vi "SensorReadMove.vi"() -> ()   [LabVIEW 2016]
uses:
  Control/Control 1.ctl
  Other Models/2010/Status/AxisDiagPacket.ctl
  Other Models/2010/Status/ControllerDiagPacket.ctl
  <vilib>/Instr/_visa.llb/VISA Configure Serial Port (Instr).vi
panel:
  in  "Speed":dbl format="%#_13g"
  in  "baud rate":u32=115200
  in  "data bits":u16=8 min=5 max=8 step=1
  in  "parity":u16(ring)=2 items=["None", "Odd", "Even", "Mark", "Space"]
  in  "stop bits":u16(ring)=10 items=["1"=10, "1.5"=15, "2.0"=20]
  in  "flow control":u16(ring) items=["None"=0, "XON/XOFF"=1, "RTS/CTS"=2, "DTR/DSR"=4]
  in  "VISA resource name":refnum<visa-resource-name>="COM4"
  out "Boolean":bool=TRUE
  in  "Iterration":i32
  in  "Input2":cluster{"X":dbl, "Y":dbl}
  in  "Input1":cluster{"X":dbl, "Y":dbl}
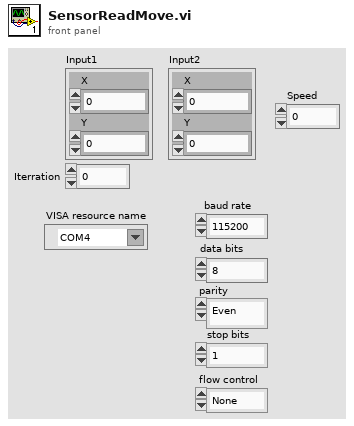
[diagram p1: front panel]
types:
  T1 = typedef "ControllerDiagPacket.ctl" = cluster{"Number of Diag Packets":i32, "Axes":T2[], "error":errorcluster}
  T2 = typedef "AxisDiagPacket.ctl" = cluster{"Axis Name":string, "Analog Input 0":dbl, "Analog Input 1":dbl, "Axis Fault (num)":i32, "Axis Fault (str)":string, "Axis Fault (bits)":cluster{"AmplifierFault":bool, "AmplifierTemperatureFault":bool, "CcwEndOfTravelLimitFault":bool, "CcwSoftwareLimitFault":bool, "CommunicationLostFault":bool, "CwEndOfTravelLimitFault":bool, "CwSoftwareLimitFault":bool, "EmergencyStopFault":bool, "EncoderFault":bool, "ExternalFault":bool, "FeedbackScalingFault":bool, "GantryMisalignFault ":bool, "HallSensorFault":bool, "InPositionTimeoutFault":bool, "InternalFault":bool, "MarkerSearchFault":bool, "MaxVelocityCommandFault":bool, "MissedInterruptFault":bool, "MotorTemperatureFault":bool, "None":bool, "OverCurrentFault":bool, "PositionErrorFault":bool, "PositionFeedbackFault":bool, "PowerSupplyFault":bool, "ProbeInputFault":bool, "SafeZoneFault":bool, "VelocityErrorFault":bool, "VelocityFeedbackFault":bool, "VoltageClampFault":bool}, "Axis Status (num)":i32, "Axis Status (str)":string, "Axis Status (bits)":cluster{"BacklashActive":bool, "CalibrationEnabled1D":bool, "CalibrationEnabled2D":bool, "CommandValid":bool, "DriveAbortPending":bool, "DrivePending":bool, "Enabling":bool, "GainMappingEnabled":bool, "GantryAligned":bool, "GantryRealigning":bool, "Homed":bool, "Homing":bool, "IFOVEnabled":bool, "JogGenerating":bool, "Jogging":bool, "JoystickControl":bool, "MasterSlaveControl":bool, "MotionBlocked":bool, "MotionClamped":bool, "MoveDone":bool, "None":bool, "NotVirtual":bool, "Profiling":bool, "Stability0":bool, "Stability1":bool, "TrajectoryFiltering":bool, "WaitDone":bool}, "Current Command":sgl, "Current Error":sgl, "Current Feedback":sgl, "Digital Inputs":i32, "Digital Outputs":i32, "Drive Status":i32, "Drive Status (str)":string, "Drive Status (bits)":cluster{"AccelerationPhase":bool, "AutofocusActive":bool, "BrakeOutput":bool, "CcwEndOfTravelLimitInput":bool, "CosineEncoderError":bool, "CurrentClamp":bool, "CwEndOfTravelLimitInput":bool, "DecelerationPhase":bool, "DualLoopActive":bool, "EmergencyStopInput":bool, "Enabled":bool, "EncoderClipping":bool, "GalvoCalibrationEnabled":bool, "GalvoPowerCorrection":bool, "HallAInput":bool, "HallBInput":bool, "HallCInput":bool, "HighResolutionMode":bool, "HomeLimitInput":bool, "InPosition":bool, "InPosition2":bool, "MarkerInput":bool, "MarkerLatch":bool, "MoveActive":bool, "NoMotorSupply":bool, "None":bool, "PowerLimiting":bool, "ProgrammingFlash":bool, "ProgrammingMXH":bool, "PSOHaltLatch":bool, "ServoControl":bool, "SineEncoderError":bool}, "Position Feedback Auxiliary":dbl, "Position Command":dbl, "Position Error":dbl, "Position Feedback":dbl, "Program Position Command":dbl, "Program Position Error":dbl, "Program Position Feedback":dbl, "Velocity Command":dbl, "Velocity Error":dbl, "Velocity Feedback":dbl}
  T3 = typedef "Control 1.ctl" = string[]
  T4 = cluster{"ControllerDiagPacket":T1, "read buffer":string}
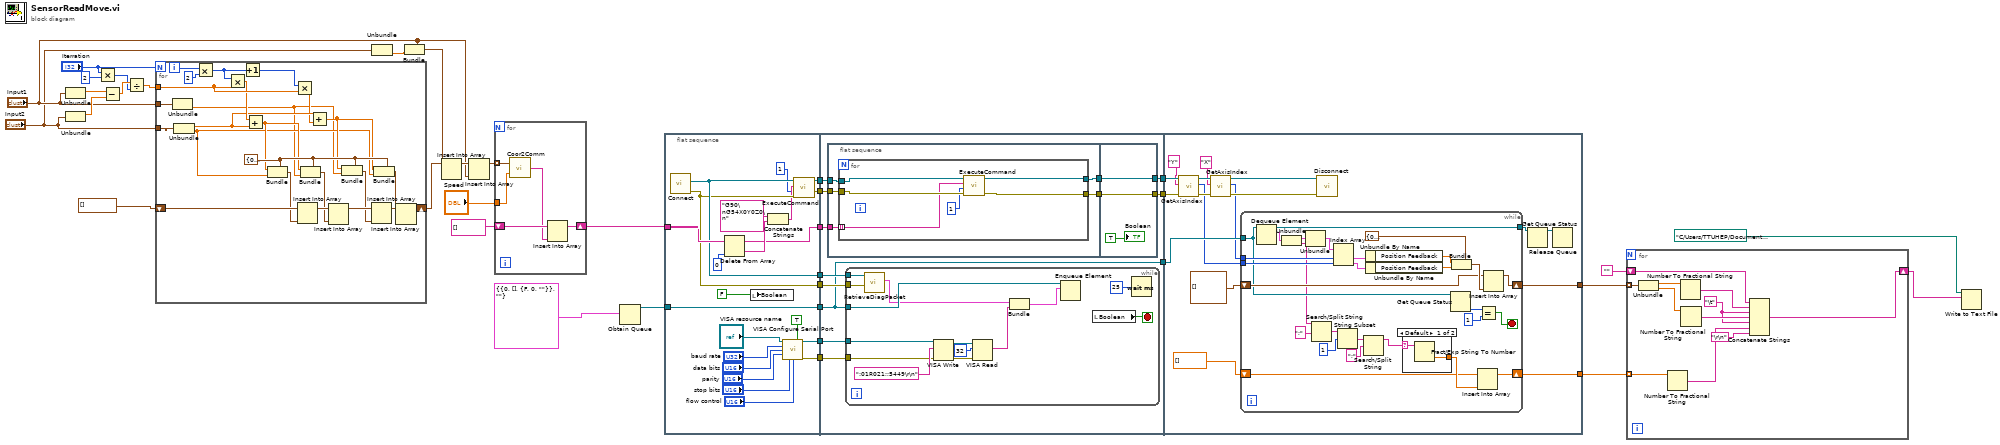
[diagram p0: block diagram]
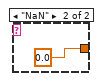
[diagram p2: hidden frame]
diagram:
  n1 = Unbundle("Input1") -> ("X"=w36:dbl)  [unwired: 1 out]
  n2 = Unbundle("Input2") -> ("X"=w35:dbl)  [unwired: 1 out]
  n3 = Multiply(x="Iterration", y=2) -> (x*y=w31:i32)
  n4 = Subtract(x=w36, y=w35) -> (x-y=w34:dbl)
  n5 = Divide(x=w34, y=w31) -> (x/y=w30:dbl)
  n6 = for {
    N: "Iterration" -> [_]
    tunnel: "Input1" -> [w49]
    tunnel: "Input2" -> [w50]
    tunnel: w30 -> [w46]
    shift-right: [w56] -> w26
    shift-left: cluster{"X":dbl, "Y":dbl}[] [] -> [w60]
    i -> [w39]
    w51 = cluster{"X":dbl, "Y":dbl} {"X"=0.0, "Y"=0.0}
    n7 = Unbundle(w49) -> ("Y"=w37:dbl)  [unwired: 1 out]
    n8 = Unbundle(w50) -> ("X"=w41:dbl, "Y"=w38:dbl)
    n9 = Multiply(x=w39, y=2) -> (x*y=w47:i32)
    n10 = Multiply(x=w47, y=w46) -> (x*y=w44:dbl)
    n11 = Increment(x=w47) -> (x+1=w45:i32)
    n12 = Add(x=w44, y=w41) -> (x+y=w43:dbl)
    n13 = Bundle(cluster=w51, "X"=w43, "Y"=w38) -> (w55:cluster{"X":dbl, "Y":dbl})
    n14 = Multiply(x=w45, y=w46) -> (x*y=w40:dbl)
    n15 = Insert Into Array(array=w60, new element=w55) -> (w59:cluster{"X":dbl, "Y":dbl}[])  [unwired: 1 in]
    n16 = Bundle(cluster=w51, "X"=w43, "Y"=w37) -> (w54:cluster{"X":dbl, "Y":dbl})
    n17 = Add(x=w41, y=w40) -> (x+y=w42:dbl)
    n18 = Insert Into Array(array=w59, new element=w54) -> (w58:cluster{"X":dbl, "Y":dbl}[])  [unwired: 1 in]
    n19 = Bundle(cluster=w51, "X"=w42, "Y"=w37) -> (w53:cluster{"X":dbl, "Y":dbl})
    n20 = Insert Into Array(array=w58, new element=w53) -> (w57:cluster{"X":dbl, "Y":dbl}[])  [unwired: 1 in]
    n21 = Bundle(cluster=w51, "X"=w42, "Y"=w38) -> (w52:cluster{"X":dbl, "Y":dbl})
    n22 = Insert Into Array(array=w57, new element=w52) -> (w56:cluster{"X":dbl, "Y":dbl}[])  [unwired: 1 in]
  }
  n23 = Unbundle("Input2") -> ("Y"=w20:dbl)  [unwired: 1 out]
  n24 = Bundle(cluster="Input1", "Y"=w20) -> (w23:cluster{"X":dbl, "Y":dbl})  [unwired: 1 in]
  n25 = Insert Into Array(array=w26, new element=w23) -> (w25:cluster{"X":dbl, "Y":dbl}[])  [unwired: 1 in]
  n26 = Insert Into Array(array=w25, new element="Input1") -> (w24:cluster{"X":dbl, "Y":dbl}[])  [unwired: 1 in]
  n27 = for {
    tunnel: w24 -> [w62] mode=indexing
    shift-right: [w64] -> w27
    shift-left: T3 [] -> [w65]
    tunnel: "Speed" -> [w61]
    n28 = call "Coor2Comm.vi"("Numeric"=w61, "Cluster"=w62) -> ("String"=w63:string)
    n29 = Insert Into Array(array=w65, new element=w63) -> (w64:T3)  [unwired: 1 in]
  }
  n30 = Obtain Queue(element data type=cluster{"ControllerDiagPacket":T1, string} {"ControllerDiagPacket"={"Number of Diag Packets"=0, "Axes"=[], "error"={"status"=FALSE, "code"=0, "source"=""}}, ""}) -> (queue out=w12:refnum<queue>)  [unwired: 4 in, 2 out]
  n31 = flat-sequence {
    tunnel: [w79] -> w17
    tunnel: [w83] -> w16
    tunnel: [w84] -> w15
    tunnel: w27 -> [w87]
    tunnel: [w86] -> w14
    tunnel: [w85] -> w13
    tunnel: w12 -> [w76]
    tunnel: [w76] -> w11
    tunnel: [w68] -> w9
    tunnel: [w67] -> w8
    tunnel: [w96] -> w19
    tunnel: [w95] -> w18
    tunnel: w17 -> [w99]
    tunnel: w16 -> [w98]
    tunnel: w15 -> [w97]
    tunnel: w14 -> [w91]
    tunnel: w13 -> [w92]
    tunnel: w11 -> [w90]
    tunnel: [w90] -> w10
    tunnel: w9 -> [w89]
    tunnel: w8 -> [w88]
    tunnel: w19 -> [w142]
    tunnel: w18 -> [w143]
    tunnel: w10 -> [w144]
    tunnel: [w129] -> w5
    tunnel: [w128] -> w6
    frame #0 {
      n32 = call "Connect.vi"() -> ("error out"=w85:errorcluster, "controller"=w86:refnum<k24>)  [unwired: 10 in]
      n33 = Delete From Array(array=w87, index=0) -> (deleted portion=w80:string, array with subset deleted=w79:T3)  [unwired: 1 in]
      n34 = local write "Boolean"(FALSE) -> ()
      n35 = Concatenate Strings("G90\nG54X0Y0Z0\n", w80) -> (w78:string)
      n36 = call-poly "VISA Configure Serial Port"("VISA resource name"="VISA resource name", "Enable Termination\nChar (T)"=TRUE, "baud rate (9600)"="baud rate", "data bits (8)"="data bits", "parity (0:none)"="parity", "stop bits (10: 1 bit)"="stop bits", "flow control (0:none)"="flow control") -> ("VISA resource name out"=w68:refnum<visa-resource-name>, "error out"=w67:errorcluster)  [unwired: 7 in]
      n37 = call "ExecuteCommand.vi"("error in (no error)"=w85, "taskId"=1, "Command Code"=w78, "controller in"=w86) -> ("error out"=w84:errorcluster, "controller out"=w83:refnum<k24>)  [unwired: 5 in, 1 out]
    }
    frame #1 {
      n38 = flat-sequence {
        tunnel: w99 -> [w118]
        tunnel: w98 -> [w117]
        tunnel: w97 -> [w116]
        tunnel: [w115] -> w94
        tunnel: [w114] -> w93
        tunnel: [w126] -> w95
        tunnel: [w127] -> w96
        tunnel: w94 -> [w127]
        tunnel: w93 -> [w126]
        frame #0 {
          n39 = for {
            tunnel: w118 -> [w122] mode=indexing
            tunnel: w117 -> [w123]
            tunnel: w116 -> [w124]
            tunnel: [w120] -> w114
            tunnel: [w119] -> w115
            n40 = call "ExecuteCommand.vi"("error in (no error)"=w124, "taskId"=1, "Command Code"=w122, "controller in"=w123) -> ("error out"=w120:errorcluster, "controller out"=w119:refnum<k24>)  [unwired: 5 in, 1 out]
          }
        }
        frame #1 {
          "Boolean" <- TRUE
        }
      }
      n41 = while {
        tunnel: w91 -> [w113]
        tunnel: w92 -> [w112]
        tunnel: w90 -> [w111]
        tunnel: w89 -> [w107]
        tunnel: w88 -> [w105]
        stop <- w109 stop-if-true
        n42 = call "RetrieveDiagPacket.vi"("error in (no error)"=w112, "Controller In"=w113) -> ("ControllerDiagPacket"=w102:T1)  [unwired: 7 in, 2 out]
        n43 = VISA Write(VISA resource name=w107, write buffer=":01R021;;5449\r\n", error in (no error)=w105) -> (VISA resource name out=w108:refnum<visa-resource-name>, error out=w104:errorcluster)  [unwired: 1 out]
        n44 = VISA Read(VISA resource name=w108, byte count=u32 32, error in (no error)=w104) -> (read buffer=w101:string)  [unwired: 3 out]
        n45 = Bundle("ControllerDiagPacket"=w102, "read buffer"=w101) -> (w100:T4)  [unwired: 1 in]
        n46 = Enqueue Element(queue=w111, element=w100) -> ()  [unwired: 2 in, 3 out]
        n47 = local read "Boolean"() -> (w109:bool)
        n48 = Wait (ms)(milliseconds to wait=25) -> ()  [unwired: 1 out]
      }
    }
    frame #2 {
      n49 = call "GetAxisIndex.vi"("error in (no error)"=w143, "axis name"="Y", "controller in"=w142) -> ("error out"=w140:errorcluster, "axis index"=w134:i32, "controller out"=w141:refnum<k24>)  [unwired: 6 in]
      n50 = call "GetAxisIndex.vi"("error in (no error)"=w140, "axis name"="X", "controller in"=w141) -> ("error out"=w139:errorcluster, "axis index"=w135:i32, "controller out"=w138:refnum<k24>)  [unwired: 6 in]
      n51 = while {
        tunnel: w135 -> [w171]
        tunnel: w134 -> [w170]
        shift-right: [w163] -> w128
        shift-left: cluster{"X":dbl, "Y":dbl}[] [] -> [w161]
        tunnel: [w162] -> w132
        tunnel: w144 -> [w157]
        shift-right: [w145] -> w129
        shift-left: dbl[] [] -> [w146]
        stop <- w159 stop-if-true
        n52 = Dequeue Element(queue=w157) -> (queue out=w162:refnum<queue>, element=w156:cluster{"ControllerDiagPacket":T1, string})  [unwired: 2 in, 2 out]
        n53 = Unbundle(w156) -> ("ControllerDiagPacket"=w155:T1, w149:string)
        n54 = Unbundle(w155) -> ("Axes"=w172:T2[])  [unwired: 2 out]
        n55 = Search/Split String(string=w149, search string/char (-)=";") -> (match + rest of string=w150:string)  [unwired: 1 in, 2 out]
        n56 = Index Array(array=w172, index #1=w171, index #2=w170) -> (element #1=w169:T2, element #2=w168:T2)
        n57 = String Subset(string=w150, offset (0)=1) -> (substring=w152:string)  [unwired: 1 in]
        n58 = Search/Split String(string=w152, search string/char (-)=";") -> (substring before match=w148:string)  [unwired: 1 in, 2 out]
        n59 = Unbundle By Name(w169) -> ("Position Feedback"=w166:dbl)
        n60 = Unbundle By Name(w168) -> ("Position Feedback"=w165:dbl)
        n61 = case shown="Default" w148 {
          selector: w148 -> [w174 _]
          tunnel: [w173 0.0] -> w147
          frame Default {
            n62 = Fract/Exp String To Number(string=w174) -> (number=w173:dbl)  [unwired: 3 in, 1 out]
          }
          frame "NaN" {
          }
        }
        n63 = Get Queue Status(queue=w157) -> (# elements in queue=w160:i32)  [unwired: 2 in, 7 out]
        n64 = Bundle(cluster=cluster{"X":dbl, "Y":dbl} {"X"=0.0, "Y"=0.0}, "X"=w166, "Y"=w165) -> (w164:cluster{"X":dbl, "Y":dbl})
        n65 = Insert Into Array(array=w146, new element=w147) -> (w145:dbl[])  [unwired: 1 in]
        n66 = Equal?(x=w160, y=1) -> (x = y?=w159:bool)
        n67 = Insert Into Array(array=w161, new element=w164) -> (w163:cluster{"X":dbl, "Y":dbl}[])  [unwired: 1 in]
      }
      n68 = call "Disconnect.vi"("error in (no error)"=w139, "controller"=w138) -> ()  [unwired: 9 in, 1 out]
      n69 = Get Queue Status(queue=w132) -> (queue out=w131:refnum<queue>)  [unwired: 2 in, 7 out]
      n70 = Release Queue(queue=w131) -> ()  [unwired: 2 in, 3 out]
    }
  }
  n71 = for {
    tunnel: w6 -> [w186] mode=indexing
    tunnel: w5 -> [w183] mode=indexing
    shift-right: [w176] -> w2
    shift-left: "" -> [w177]
    w179 = "\t"
    n72 = Unbundle(w186) -> ("X"=w185:dbl, "Y"=w184:dbl)
    n73 = Number To Fractional String(number=w183) -> (F-format string=w180:string)  [unwired: 3 in]
    n74 = Number To Fractional String(number=w185) -> (F-format string=w182:string)  [unwired: 3 in]
    n75 = Number To Fractional String(number=w184) -> (F-format string=w181:string)  [unwired: 3 in]
    n76 = Concatenate Strings(w177, w182, w179, w181, w179, w180, "\r\n") -> (w176:string)
  }
  n77 = Write to Text File(file (use dialog)=path "C:/Users/TTUHEP/Documents/LabVIEW/output.txt", text=w2) -> ()  [unwired: 2 in, 3 out]
